vi "Guardadoarreglosmult.vi"(4 "disp 3":dbl[][][][][](array[numeric]), 5 "disp 1":dbl[][][](array[numeric]), 6 "disp 2":dbl[][][][](array[numeric]), 7 "disp 0":dbl[][](array[numeric]), 9 "Enum":T1(ring), 10 "indice":i32, 11 "nombre":string) -> ()   [LabVIEW 2016]
uses:
  <vilib>/UPVI/lvhdf5/file.llb/LVH5F Operation.ctl
  <vilib>/Utility/miscctls.llb/LVRectTypeDef.ctl
  <vilib>/UPVI/lvhdf5/group.llb/H5G_obj_t.ctl
  <vilib>/UPVI/lvhdf5/dataset.llb/LVH5D Operation.ctl
  <vilib>/UPVI/lvhdf5/group.llb/OpenCreateGroup (String).vi
  <vilib>/UPVI/lvhdf5/utility.llb/Select HDF5 Dialog.vi
  <vilib>/UPVI/lvhdf5/utility.llb/Select HDF5 Dialog (Object Only).vi
  <vilib>/UPVI/lvhdf5/dataset.llb/Simple H5Dwrite (Variant).vi
  <vilib>/UPVI/lvhdf5/dataset.llb/Simple H5Dwrite.xnode
  <vilib>/UPVI/lvhdf5/library.llb/HDF5 Ref.ctl
  <vilib>/UPVI/lvhdf5/identifier.llb/Not an HDF5 Refnum Constant.vi
  <vilib>/Utility/error.llb/Error Cluster From Error Code.vi
  <vilib>/UPVI/lvhdf5/dataset.llb/OpenCreateReplace Dataset by Element Type.vi
  <vilib>/UPVI/lvhdf5/dataspace.llb/H5Sselect_hyperslab.vi
  <vilib>/UPVI/lvhdf5/dataset.llb/H5Dwrite (Variant).vi
  <vilib>/UPVI/lvhdf5/dataset.llb/H5Dget_space.vi
  <vilib>/UPVI/lvhdf5/attribute.llb/private/LVH5AwriteWDTAttrs.vi
  <vilib>/UPVI/lvhdf5/dataspace.llb/H5Sclose.vi
  <vilib>/UPVI/lvhdf5/dataset.llb/H5Dclose.vi
  <vilib>/UPVI/lvhdf5/utility.llb/Select HDF5 Dialog (File and Object).vi
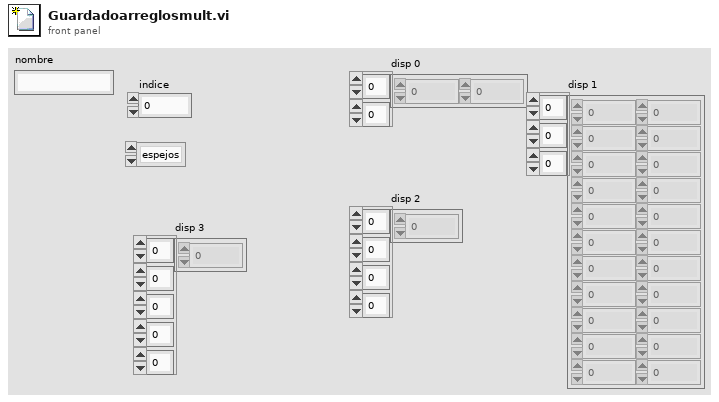
[diagram p1: front panel]
types:
  T1 = enum16{"espejos", "polarizador", "voltaje", "potenciometro ", "CCD", "lockin", "laser", "multimetro", "ninguno"}
  T2 = typedef "LVH5F Operation.ctl" = enum16{"open", "open or create", "create or replace", "create or replace (with confirmation)", "create", "open (read only)"}
  T3 = typedef "HDF5 Ref.ctl" = refnum<k1>
  T4 = typedef "LVRectTypeDef.ctl" = cluster{"Left":i16, "Top":i16, "Right":i16, "Bottom":i16}
  T5 = cluster{"Behavior":enum32{"Invalid", "Default", "Floating", "Floating/Auto-Hide", "Modal"}, "Position":T4, "Center":bool, "Title":string}
  T6 = typedef "LVH5D Operation.ctl" = enum16{"open", "replace", "create", "open or create", "create or replace", "create or replace with confirmation"}
  T7 = typedef "H5G_obj_t.ctl" = i32
  T8 = cluster{"Object Types (any)":T7[], "Object Pattern":string}
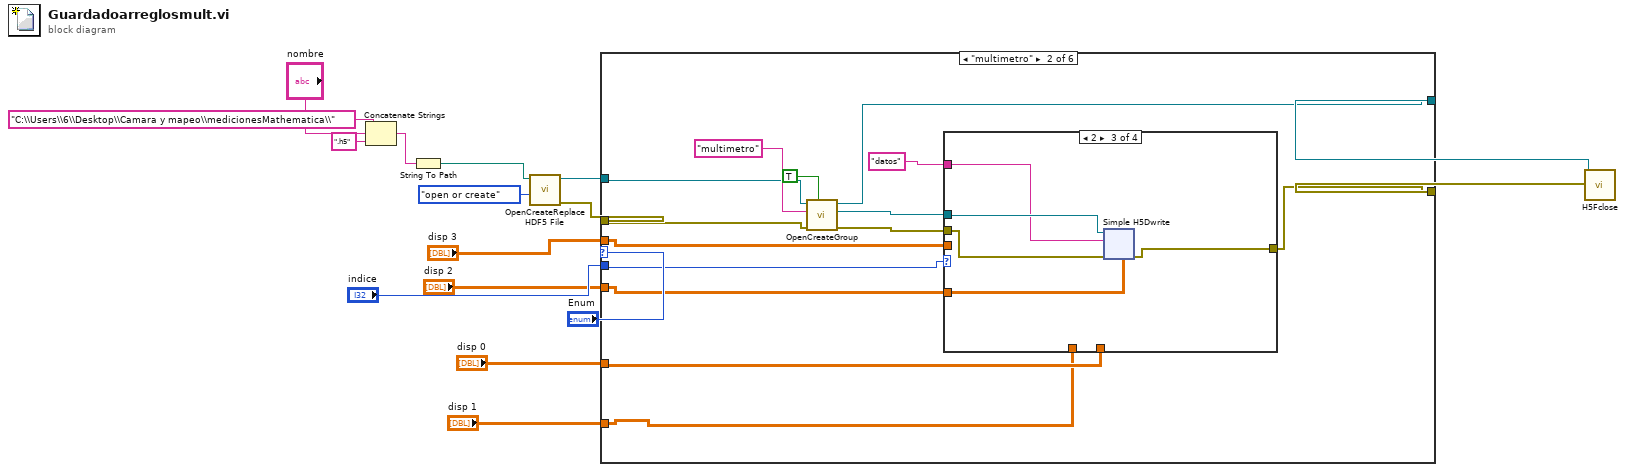
[diagram p0: block diagram]
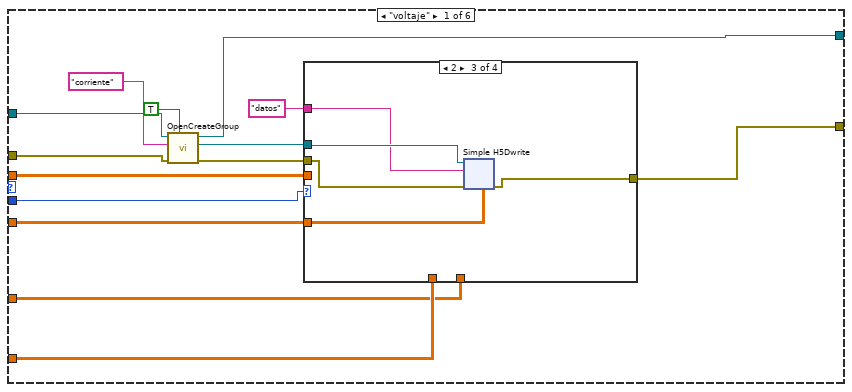
[diagram p2: hidden frame]
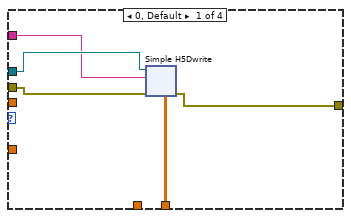
[diagram p3: hidden frame]
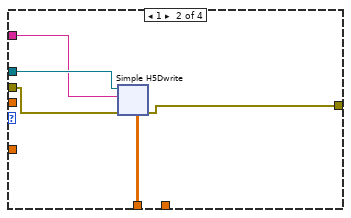
[diagram p4: hidden frame]
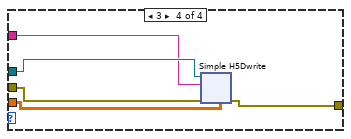
[diagram p5: hidden frame]
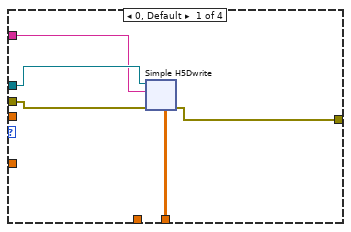
[diagram p6: hidden frame]
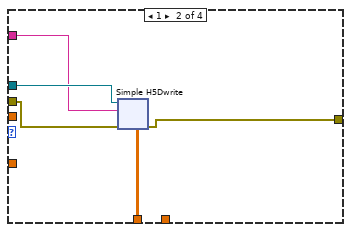
[diagram p7: hidden frame]
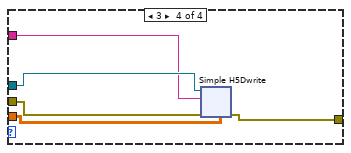
[diagram p8: hidden frame]
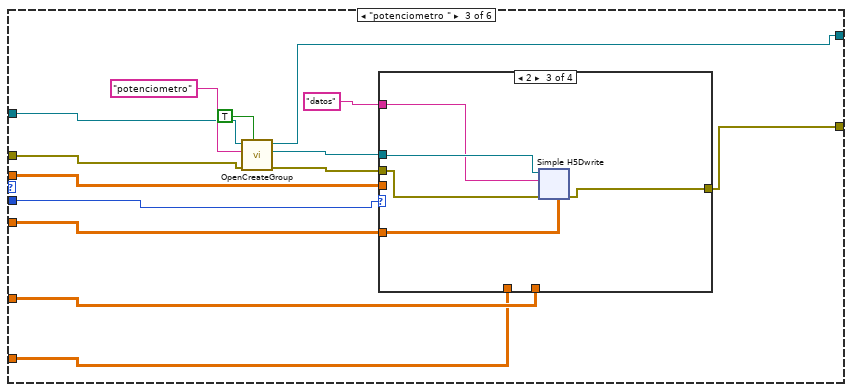
[diagram p9: hidden frame]
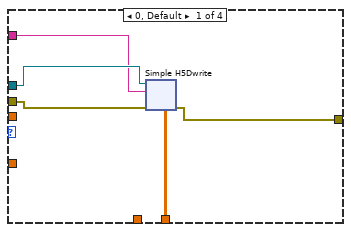
[diagram p10: hidden frame]
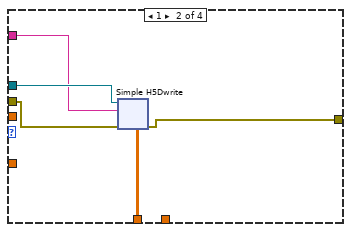
[diagram p11: hidden frame]
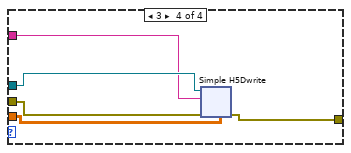
[diagram p12: hidden frame]
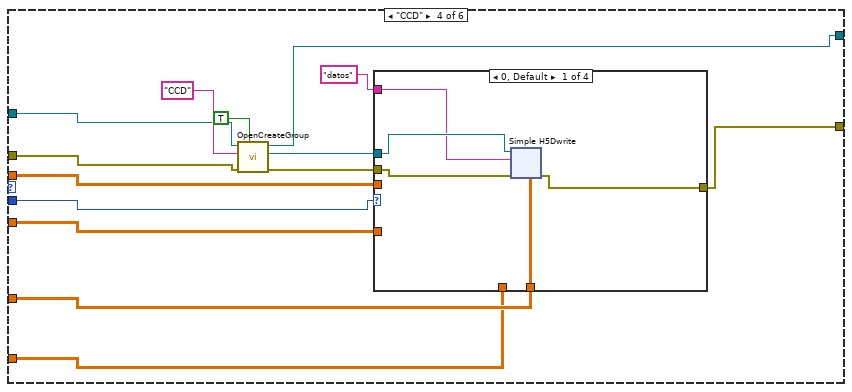
[diagram p13: hidden frame]
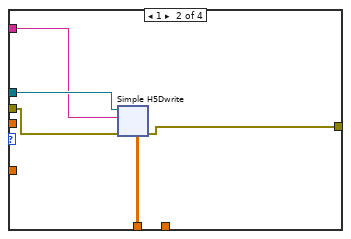
[diagram p14: hidden frame]
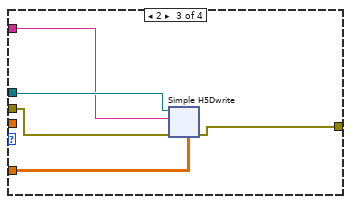
[diagram p15: hidden frame]
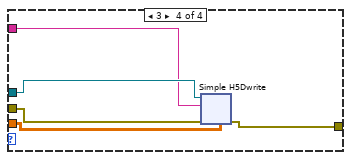
[diagram p16: hidden frame]
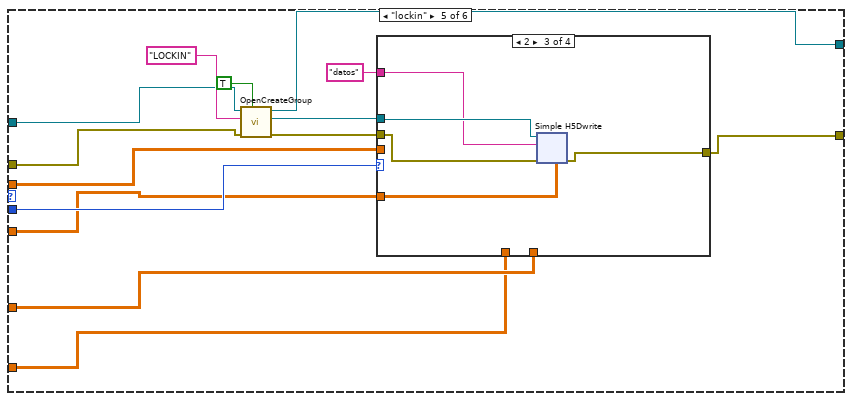
[diagram p17: hidden frame]
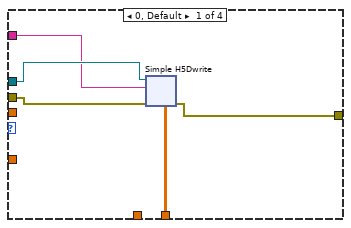
[diagram p18: hidden frame]
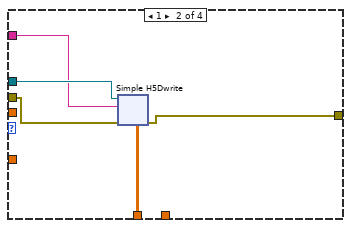
[diagram p19: hidden frame]
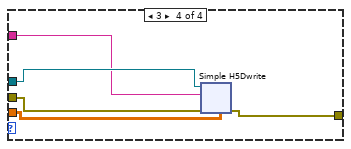
[diagram p20: hidden frame]
diagram:
  n1 = Concatenate Strings("C:\\Users\\6\\Desktop\\Camara y mapeo\\medicionesMathematica\\" ("string"), "nombre", ".h5" ("string")) -> (w13:string)
  n2 = String To Path(string=w13) -> (path=w12:path)
  n3 = call <vilib>:"OpenCreateReplace HDF5 File.vi"("function (open or create)"=LVH5F_Operation."open or create", "path"=w12) -> ("error out"=w7:errorcluster, "HDF5 Ref out"=w8:T3)  [unwired: 6 in]
  n4 = case shown="\"multimetro\"" "Enum" {
    tunnel: "indice" -> [w30 w859 w1707 w2550 w3391 _]
    tunnel: w8 -> [w29 w865 w1711 w2553 w3394 w4228]
    tunnel: w7 -> [w24 w864 w1709 w2552 w3393 w4227]
    tunnel: [w26 w867 w1710 w2546 w3395 w4228] -> w2
    tunnel: "disp 1" -> [w23 w860 w1704 w2547 w3388 _]
    tunnel: "disp 0" -> [w22 w861 w1705 w2548 w3389 _]
    tunnel: "disp 2" -> [w21 w862 w1706 w2549 w3390 _]
    tunnel: "disp 3" -> [w20 w863 w1708 w2551 w3392 _]
    tunnel: [w19 w866 w1703 w2545 w3387 w4227] -> w1
    frame "voltaje" {
      n5 = call-poly <vilib>:"OpenCreateGroup.vi"("Create if not found (F)"=TRUE, "error in (no error)"=w24, "Group"="corriente", "HDF5 Ref"=w29) -> ("error out"=w25:errorcluster, "HDF5 Group Ref"=w27:T3, "HDF5 Ref out"=w26:T3)  [unwired: 5 in]
      n6 = case shown="2" w30 {
        tunnel: w27 -> [w35 w242 w449 w656]
        tunnel: w25 -> [w34 w241 w448 w655]
        tunnel: w23 -> [_ w240 _ _]
        tunnel: w22 -> [w33 _ _ _]
        tunnel: w21 -> [_ _ w447 _]
        tunnel: w20 -> [_ _ _ w654]
        tunnel: [w32 w239 w446 w653] -> w19
        tunnel: "datos" ("Dataset Path") -> [w31 w238 w445 w652]
        frame 0, Default {
          n7 = xnode "Simple H5Dwrite"("Dataset Path"=w31, "error in (no error)"=w34, "HDF5 Path or Ref"=w35, "Data"=w33) -> ("error out"=w32:errorcluster)  [unwired: 4 in, 2 out]
        }
        frame 1 {
          n8 = xnode "Simple H5Dwrite"("Dataset Path"=w238, "error in (no error)"=w241, "HDF5 Path or Ref"=w242, "Data"=w240) -> ("error out"=w239:errorcluster)  [unwired: 4 in, 2 out]
        }
        frame 2 {
          n9 = xnode "Simple H5Dwrite"("Dataset Path"=w445, "error in (no error)"=w448, "HDF5 Path or Ref"=w449, "Data"=w447) -> ("error out"=w446:errorcluster)  [unwired: 4 in, 2 out]
        }
        frame 3 {
          n10 = xnode "Simple H5Dwrite"("Dataset Path"=w652, "error in (no error)"=w655, "HDF5 Path or Ref"=w656, "Data"=w654) -> ("error out"=w653:errorcluster)  [unwired: 4 in, 2 out]
        }
      }
    }
    frame "multimetro" {
      n11 = call-poly <vilib>:"OpenCreateGroup.vi"("Create if not found (F)"=TRUE, "error in (no error)"=w864, "Group"="multimetro", "HDF5 Ref"=w865) -> ("error out"=w870:errorcluster, "HDF5 Group Ref"=w871:T3, "HDF5 Ref out"=w867:T3)  [unwired: 5 in]
      n12 = case shown="2" w859 {
        tunnel: w871 -> [w877 w1084 w1291 w1498]
        tunnel: w870 -> [w876 w1083 w1290 w1497]
        tunnel: w860 -> [_ w1082 _ _]
        tunnel: w861 -> [w875 _ _ _]
        tunnel: w862 -> [_ _ w1289 _]
        tunnel: w863 -> [_ _ _ w1496]
        tunnel: [w874 w1081 w1288 w1495] -> w866
        tunnel: "datos" ("Dataset Path") -> [w873 w1080 w1287 w1494]
        frame 0, Default {
          n13 = xnode "Simple H5Dwrite"("Dataset Path"=w873, "error in (no error)"=w876, "HDF5 Path or Ref"=w877, "Data"=w875) -> ("error out"=w874:errorcluster)  [unwired: 4 in, 2 out]
        }
        frame 1 {
          n14 = xnode "Simple H5Dwrite"("Dataset Path"=w1080, "error in (no error)"=w1083, "HDF5 Path or Ref"=w1084, "Data"=w1082) -> ("error out"=w1081:errorcluster)  [unwired: 4 in, 2 out]
        }
        frame 2 {
          n15 = xnode "Simple H5Dwrite"("Dataset Path"=w1287, "error in (no error)"=w1290, "HDF5 Path or Ref"=w1291, "Data"=w1289) -> ("error out"=w1288:errorcluster)  [unwired: 4 in, 2 out]
        }
        frame 3 {
          n16 = xnode "Simple H5Dwrite"("Dataset Path"=w1494, "error in (no error)"=w1497, "HDF5 Path or Ref"=w1498, "Data"=w1496) -> ("error out"=w1495:errorcluster)  [unwired: 4 in, 2 out]
        }
      }
    }
    frame "potenciometro " {
      n17 = call-poly <vilib>:"OpenCreateGroup.vi"("Create if not found (F)"=TRUE, "error in (no error)"=w1709, "Group"="potenciometro", "HDF5 Ref"=w1711) -> ("error out"=w1712:errorcluster, "HDF5 Group Ref"=w1713:T3, "HDF5 Ref out"=w1710:T3)  [unwired: 5 in]
      n18 = case shown="2" w1707 {
        tunnel: w1713 -> [w1719 w1926 w2133 w2340]
        tunnel: w1712 -> [w1718 w1925 w2132 w2339]
        tunnel: w1704 -> [_ w1924 _ _]
        tunnel: w1705 -> [w1717 _ _ _]
        tunnel: w1706 -> [_ _ w2131 _]
        tunnel: w1708 -> [_ _ _ w2338]
        tunnel: [w1716 w1923 w2130 w2337] -> w1703
        tunnel: "datos" ("Dataset Path") -> [w1715 w1922 w2129 w2336]
        frame 0, Default {
          n19 = xnode "Simple H5Dwrite"("Dataset Path"=w1715, "error in (no error)"=w1718, "HDF5 Path or Ref"=w1719, "Data"=w1717) -> ("error out"=w1716:errorcluster)  [unwired: 4 in, 2 out]
        }
        frame 1 {
          n20 = xnode "Simple H5Dwrite"("Dataset Path"=w1922, "error in (no error)"=w1925, "HDF5 Path or Ref"=w1926, "Data"=w1924) -> ("error out"=w1923:errorcluster)  [unwired: 4 in, 2 out]
        }
        frame 2 {
          n21 = xnode "Simple H5Dwrite"("Dataset Path"=w2129, "error in (no error)"=w2132, "HDF5 Path or Ref"=w2133, "Data"=w2131) -> ("error out"=w2130:errorcluster)  [unwired: 4 in, 2 out]
        }
        frame 3 {
          n22 = xnode "Simple H5Dwrite"("Dataset Path"=w2336, "error in (no error)"=w2339, "HDF5 Path or Ref"=w2340, "Data"=w2338) -> ("error out"=w2337:errorcluster)  [unwired: 4 in, 2 out]
        }
      }
    }
    frame "CCD" {
      n23 = call-poly <vilib>:"OpenCreateGroup.vi"("Create if not found (F)"=TRUE, "error in (no error)"=w2552, "Group"="CCD", "HDF5 Ref"=w2553) -> ("error out"=w2554:errorcluster, "HDF5 Group Ref"=w2555:T3, "HDF5 Ref out"=w2546:T3)  [unwired: 5 in]
      n24 = case shown="0, Default" w2550 {
        tunnel: w2555 -> [w2561 w2768 w2975 w3182]
        tunnel: w2554 -> [w2560 w2767 w2974 w3181]
        tunnel: w2547 -> [_ w2766 _ _]
        tunnel: w2548 -> [w2559 _ _ _]
        tunnel: w2549 -> [_ _ w2973 _]
        tunnel: w2551 -> [_ _ _ w3180]
        tunnel: [w2558 w2765 w2972 w3179] -> w2545
        tunnel: "datos" ("Dataset Path") -> [w2557 w2764 w2971 w3178]
        frame 0, Default {
          n25 = xnode "Simple H5Dwrite"("Dataset Path"=w2557, "error in (no error)"=w2560, "HDF5 Path or Ref"=w2561, "Data"=w2559) -> ("error out"=w2558:errorcluster)  [unwired: 4 in, 2 out]
        }
        frame 1 {
          n26 = xnode "Simple H5Dwrite"("Dataset Path"=w2764, "error in (no error)"=w2767, "HDF5 Path or Ref"=w2768, "Data"=w2766) -> ("error out"=w2765:errorcluster)  [unwired: 4 in, 2 out]
        }
        frame 2 {
          n27 = xnode "Simple H5Dwrite"("Dataset Path"=w2971, "error in (no error)"=w2974, "HDF5 Path or Ref"=w2975, "Data"=w2973) -> ("error out"=w2972:errorcluster)  [unwired: 4 in, 2 out]
        }
        frame 3 {
          n28 = xnode "Simple H5Dwrite"("Dataset Path"=w3178, "error in (no error)"=w3181, "HDF5 Path or Ref"=w3182, "Data"=w3180) -> ("error out"=w3179:errorcluster)  [unwired: 4 in, 2 out]
        }
      }
    }
    frame "lockin" {
      n29 = call-poly <vilib>:"OpenCreateGroup.vi"("Create if not found (F)"=TRUE, "error in (no error)"=w3393, "Group"="LOCKIN", "HDF5 Ref"=w3394) -> ("error out"=w3396:errorcluster, "HDF5 Group Ref"=w3397:T3, "HDF5 Ref out"=w3395:T3)  [unwired: 5 in]
      n30 = case shown="2" w3391 {
        tunnel: w3397 -> [w3403 w3610 w3817 w4024]
        tunnel: w3396 -> [w3402 w3609 w3816 w4023]
        tunnel: w3388 -> [_ w3608 _ _]
        tunnel: w3389 -> [w3401 _ _ _]
        tunnel: w3390 -> [_ _ w3815 _]
        tunnel: w3392 -> [_ _ _ w4022]
        tunnel: [w3400 w3607 w3814 w4021] -> w3387
        tunnel: "datos" ("Dataset Path") -> [w3399 w3606 w3813 w4020]
        frame 0, Default {
          n31 = xnode "Simple H5Dwrite"("Dataset Path"=w3399, "error in (no error)"=w3402, "HDF5 Path or Ref"=w3403, "Data"=w3401) -> ("error out"=w3400:errorcluster)  [unwired: 4 in, 2 out]
        }
        frame 1 {
          n32 = xnode "Simple H5Dwrite"("Dataset Path"=w3606, "error in (no error)"=w3609, "HDF5 Path or Ref"=w3610, "Data"=w3608) -> ("error out"=w3607:errorcluster)  [unwired: 4 in, 2 out]
        }
        frame 2 {
          n33 = xnode "Simple H5Dwrite"("Dataset Path"=w3813, "error in (no error)"=w3816, "HDF5 Path or Ref"=w3817, "Data"=w3815) -> ("error out"=w3814:errorcluster)  [unwired: 4 in, 2 out]
        }
        frame 3 {
          n34 = xnode "Simple H5Dwrite"("Dataset Path"=w4020, "error in (no error)"=w4023, "HDF5 Path or Ref"=w4024, "Data"=w4022) -> ("error out"=w4021:errorcluster)  [unwired: 4 in, 2 out]
        }
      }
    }
    frame "ninguno", Default {
    }
  }
  n35 = call <vilib>:"H5Fclose.vi"("error in (no error)"=w1, "HDF5 Ref"=w2) -> ()  [unwired: 7 in, 1 out]
